vi "Set Robot Position.vi"(5 "Goal":cluster{"X":dbl, "Y":dbl}, 6 "Wheel theta":dbl[](array[numeric])=[200.0, -200.0, -200.0, 200.0], 7 "Odometry Data":dbl[](array[numeric]), 8 "error in (no error)":errorcluster, 9 "axles":refnum<vi>[](array[refnum]), 10 "robot":refnum<vi>, 11 "scene in":refnum<vi>) -> (0 "error out":errorcluster, 3 "scene out":refnum<vi>)   [LabVIEW 2017]
uses:
  <vilib>/picture/3D Picture Control/NI_3D Picture Control.lvlib
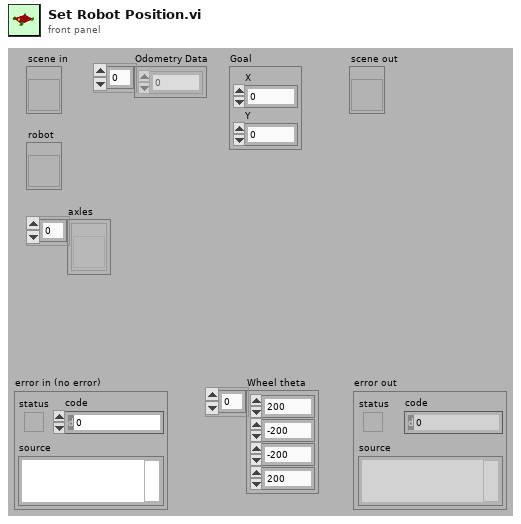
[diagram p1: front panel]
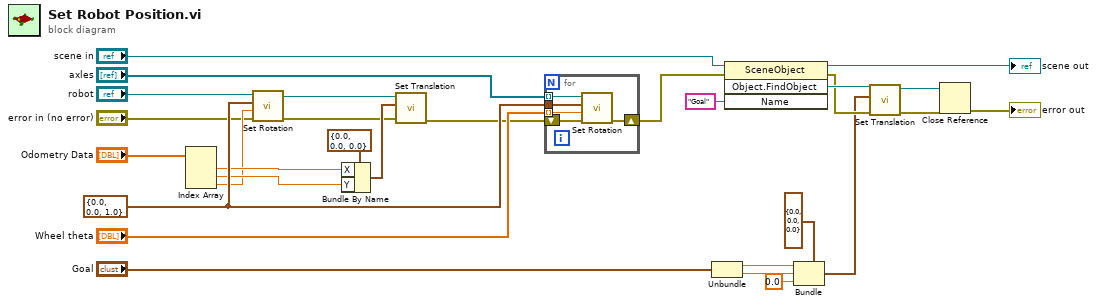
[diagram p0: block diagram]
diagram:
  w26 = cluster{"X":sgl, "Y":sgl, "Z":sgl} {"X"=0.0, "Y"=0.0, "Z"=1.0} ("Axis")
  n1 = Index Array(array="Odometry Data") -> (element #1=w24:dbl, element #2=w23:dbl, element #3=w6:dbl)  [unwired: 3 in]
  n2 = call <vilib>:"Set Rotation.vi"("error in (no error)"="error in (no error)", "Angle"=w6, "Axis"=w26, "Scene Object"="robot") -> ("error out"=w3:errorcluster, "Rotated Scene Object"=w21:refnum<vi>)  [unwired: 6 out]
  n3 = Bundle By Name(cluster=cluster{"X":sgl, "Y":sgl, "Z":sgl} {"X"=0.0, "Y"=0.0, "Z"=0.0} ("Axis"), "X"=w24, "Y"=w23) -> (w22:cluster{"X":sgl, "Y":sgl, "Z":sgl})
  n4 = call <vilib>:"Set Translation.vi"("error in (no error)"=w3, "Translation"=w22, "Scene Object"=w21) -> ("error out"=w2:errorcluster)  [unwired: 8 out]
  n5 = for {
    tunnel: "axles" -> [w33] mode=indexing
    tunnel: w26 -> [w34]
    tunnel: "Wheel theta" -> [w32] mode=indexing
    shift-right: [w31] -> w1
    shift-left: w2 -> [w30]
    n6 = call <vilib>:"Set Rotation.vi"("error in (no error)"=w30, "Angle"=w32, "Axis"=w34, "Scene Object"=w33) -> ("error out"=w31:errorcluster)  [unwired: 7 out]
  }
  n7 = Unbundle("Goal") -> ("X"=w11:dbl, "Y"=w10:dbl)
  n8 = invoke class="SceneObject" method="Object.FindObject"(reference="scene in", error in=w1, "Name"="Goal") -> (reference out=→"scene out":refnum<vi>, error out=w15:errorcluster, "FindObject"=w17:refnum<vi>)  [unwired: 1 in, 1 out]
  n9 = Bundle(cluster=cluster{"X":sgl, "Y":sgl, "Z":sgl} {"X"=0.0, "Y"=0.0, "Z"=0.0} ("Translation"), "X"=w11, "Y"=w10, "Z"=sgl 0.0) -> (w8:cluster{"X":sgl, "Y":sgl, "Z":sgl})
  n10 = call <vilib>:"Set Translation.vi"("error in (no error)"=w15, "Translation"=w8, "Scene Object"=w17) -> ("error out"=w14:errorcluster, "Translated Object"=w16:refnum<vi>)  [unwired: 7 out]
  n11 = Close Reference(reference=w16, error in (no error)=w14) -> (error out=→"error out":errorcluster)
